vi "Read Measurement (2 Channels).vi"(6 "Measurement Type (0: Phase)":i32(ring) items=["Phase", "Delay", "DelayRR", "DelayRF", "DelayFR", "DelayFF"], 8 "error in (no error)":errorcluster, 9 "Channel 2 (2: Channel 2)":i32(ring)=2 items=["Channel 1"=1, "Channel 2"=2, "Channel 3"=3, "Channel 4"=4], 10 "Channel 1 (1: Channel 1)":i32(ring)=1 items=["Channel 1"=1, "Channel 2"=2, "Channel 3"=3, "Channel 4"=4], 11 "VISA resource name":refnum<visa-resource-name>) -> (0 "error out":errorcluster, 1 "Units":string, 2 "Measurement":dbl, 3 "VISA resource name out":refnum<visa-resource-name>)   [LabVIEW 2012, in "Tektronix TDS 200 1000 2000 Series.lvlib"]
doc: "This VI displays the results of the selected 2 channels measurement."
uses:
  <instrlib>/Tektronix TDS 200 1000 2000 Series/Tektronix TDS 200 1000 2000 Series.lvlib
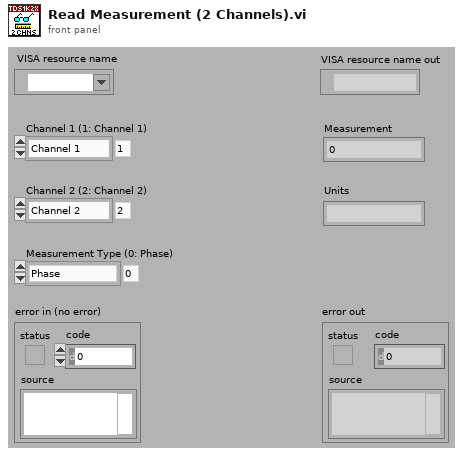
[diagram p1: front panel]
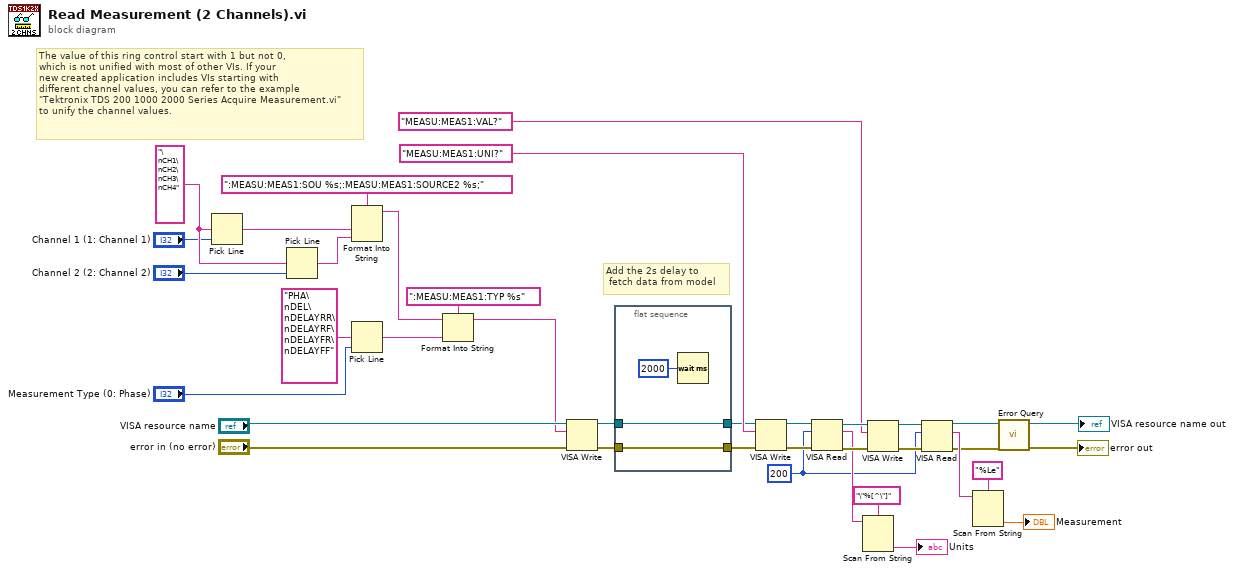
[diagram p0: block diagram]
diagram:
  w1 = u32 200 ("byte count")
  w20 = "\nCH1\nCH2\nCH3\nCH4"
  # "The value of this ring control start with 1 but not 0, \nwhich is not unified with most of other VIs. If your \nnew created application includes VIs starting with \ndifferent channel values, you can refer to the example\n\"Tektronix TDS 200 1000 2000 Series Acquire Measurement.vi\"\nto unify the channel values."
  # "Add the 2s delay to\n fetch data from model"
  n1 = Pick Line(multi-line string=w20, line index="Channel 1 (1: Channel 1)") -> (output string=w18:string)  [unwired: 1 out]
  n2 = Pick Line(multi-line string=w20, line index="Channel 2 (2: Channel 2)") -> (output string=w19:string)  [unwired: 1 out]
  n3 = Format Into String(format string=":MEASU:MEAS1:SOU %s;:MEASU:MEAS1:SOURCE2 %s;", w18, w19) -> (resulting string=w4:string)  [unwired: 2 in, 1 out]
  n4 = Pick Line(multi-line string="PHA\nDEL\nDELAYRR\nDELAYRF\nDELAYFR\nDELAYFF", line index="Measurement Type (0: Phase)") -> (output string=w6:string)  [unwired: 1 out]
  n5 = Format Into String(format string=":MEASU:MEAS1:TYP %s", initial string=w4, w6) -> (resulting string=w3:string)  [unwired: 1 in, 1 out]
  n6 = VISA Write(VISA resource name="VISA resource name", write buffer=w3, error in (no error)="error in (no error)") -> (VISA resource name out=w11:refnum<visa-resource-name>, error out=w10:errorcluster)  [unwired: 1 out]
  n7 = flat-sequence {
    tunnel: w11 -> [w39]
    tunnel: w10 -> [w40]
    tunnel: [w40] -> w9
    tunnel: [w39] -> w8
    frame #0 {
      n8 = Wait (ms)(milliseconds to wait=u32 2000) -> ()  [unwired: 1 out]
    }
  }
  n9 = VISA Write(VISA resource name=w8, write buffer="MEASU:MEAS1:UNI?", error in (no error)=w9) -> (VISA resource name out=w37:refnum<visa-resource-name>, error out=w36:errorcluster)  [unwired: 1 out]
  n10 = VISA Read(VISA resource name=w37, byte count=w1, error in (no error)=w36) -> (VISA resource name out=w32:refnum<visa-resource-name>, read buffer=w27:string, error out=w31:errorcluster)  [unwired: 1 out]
  n11 = Scan From String(format string="\"%[^\"]", input string=w27) -> (output 1=→"Units":string)  [unwired: 2 in, 4 out]
  n12 = VISA Write(VISA resource name=w32, write buffer="MEASU:MEAS1:VAL?", error in (no error)=w31) -> (VISA resource name out=w34:refnum<visa-resource-name>, error out=w33:errorcluster)  [unwired: 1 out]
  n13 = VISA Read(VISA resource name=w34, byte count=w1, error in (no error)=w33) -> (VISA resource name out=w15:refnum<visa-resource-name>, read buffer=w29:string, error out=w14:errorcluster)  [unwired: 1 out]
  n14 = Scan From String(format string="%Le", input string=w29) -> (output 1=→"Measurement":dbl)  [unwired: 2 in, 4 out]
  n15 = call <instrlib>:"Error Query.vi"("error in (no error)"=w14, "VISA resource name"=w15) -> ("error out"=→"error out":errorcluster, "VISA resource name out"=→"VISA resource name out":refnum<visa-resource-name>)  [unwired: 8 out]
